vi "speedmode.vi"(6 "offset X":dbl, 7 "offset Y":dbl, 9 "beamsize x tolerance":dbl, 10 "Speedmode @":dbl, 11 "step size":dbl) -> (1 "steps speed Y":dbl, 2 "steps speed X":dbl, 3 "speedmode X":bool, 4 "speedmode Y":bool)   [LabVIEW 2020]
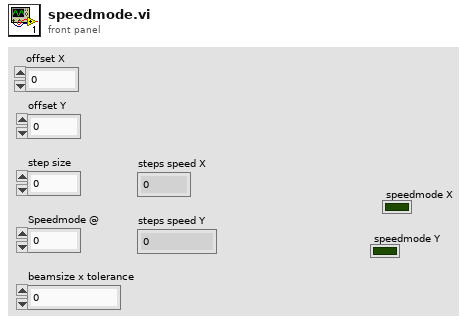
[diagram p1: front panel]
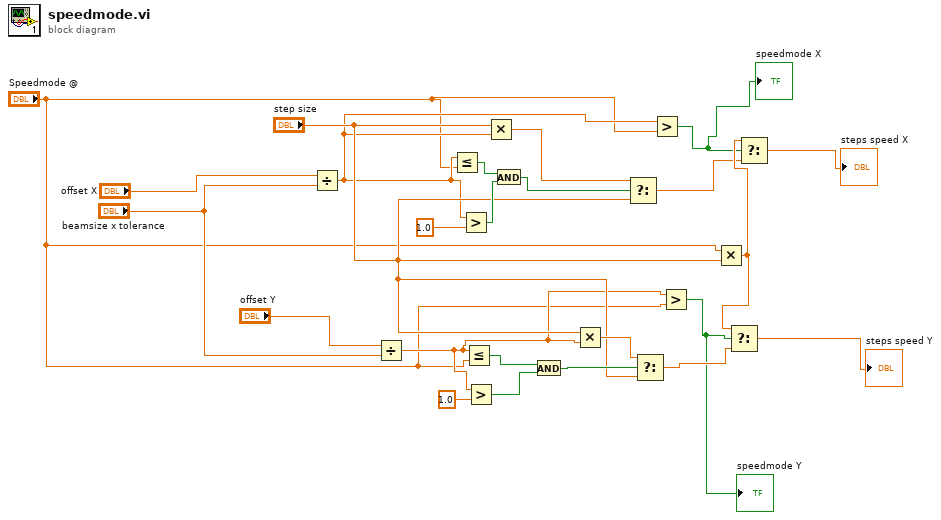
[diagram p0: block diagram]
diagram:
  n1 = Divide(x="offset X", y="beamsize x tolerance") -> (x/y=w6:dbl)
  n2 = Divide(x="offset Y", y="beamsize x tolerance") -> (x/y=w7:dbl)
  n3 = Less Or Equal?(x=w6, y="Speedmode @") -> (x <= y?=w16:bool)
  n4 = Greater?(x=w6, y=1.0) -> (0:w15:bool)
  n5 = Less Or Equal?(x=w7, y="Speedmode @") -> (x <= y?=w21:bool)
  n6 = Greater?(x=w7, y=1.0) -> (0:w20:bool)
  n7 = Multiply(x="step size", y=w6) -> (x*y=w18:dbl)
  n8 = And(x=w16, y=w15) -> (x .and. y?=w17:bool)
  n9 = And(x=w21, y=w20) -> (x .and. y?=w22:bool)
  n10 = Multiply(x="step size", y=w7) -> (x*y=w23:dbl)
  n11 = Select(t=w18, s=w17, f="step size") -> (s? t:f=w3:dbl)
  n12 = Select(t=w23, s=w22, f="step size") -> (s? t:f=w10:dbl)
  n13 = Greater?(x=w6, y="Speedmode @") -> (0:w1:bool)
  "speedmode X" <- w1
  n14 = Greater?(x=w7, y="Speedmode @") -> (0:w8:bool)
  "speedmode Y" <- w8
  n15 = Multiply(x="Speedmode @", y="step size") -> (x*y=w4:dbl)
  n16 = Select(t=w4, s=w8, f=w10) -> (s? t:f=→"steps speed Y":dbl)
  n17 = Select(t=w4, s=w1, f=w3) -> (s? t:f=→"steps speed X":dbl)
